vi "Configure Command Format.vi"(0 "VISA resource name":refnum<visa-resource-name>, 7 "Command format (T: Byte)":bool=TRUE, 11 "error in (no error)":errorcluster) -> (4 "VISA resource name out":refnum<visa-resource-name>, 15 "error out":errorcluster)   [LabVIEW 2020, in "LeCroy Wave Series.lvlib"]
doc: "Selects the format the oscilloscope uses to send waveform data."
uses:
  LeCroy Wave Series.lvlib
panel:
  # "Byte"
  # "Word"
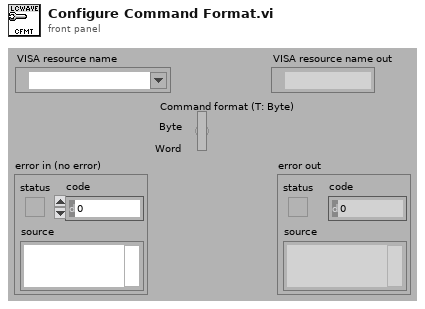
[diagram p1: front panel]
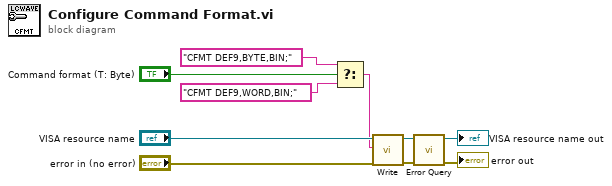
[diagram p0: block diagram]
diagram:
  n1 = Select(t="CFMT DEF9,BYTE,BIN;", s="Command format (T: Byte)", f="CFMT DEF9,WORD,BIN;") -> (s? t:f=w5:string)
  n2 = call "Write.vi"("error in (no error)"="error in (no error)", "Write Buffer"=w5, "VISA resource name"="VISA resource name") -> ("error out"=w1:errorcluster, "VISA resource name out"=w4:refnum<visa-resource-name>)  [unwired: 6 in, 1 out]
  n3 = call "Error Query.vi"("error in (no error)"=w1, "VISA resource name"=w4) -> ("error out"=→"error out":errorcluster, "VISA resource name out"=→"VISA resource name out":refnum<visa-resource-name>)  [unwired: 6 in, 2 out]
